vi "Compact.vi"(1 "bytestream":refnum<class "Bytestream.lvclass">) -> (0 "bytestream out":refnum<class "Bytestream.lvclass">)   [LabVIEW 2020, in "NI_Bytestream.lvlib" / "Bytestream.lvclass"]
uses:
  <vilib>/Array/Bytestream/Bytestream.lvclass
  <vilib>/Array/Bytestream/Bytestream.lvclass/Bytestream.ctl
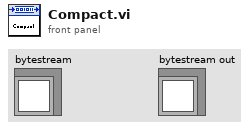
[diagram p1: front panel]
types:
  T1 = typedef "NI_Bytestream.lvlib/Bytestream.lvclass/Datum.ctl" = cluster{"array":u8[], "index":i32}
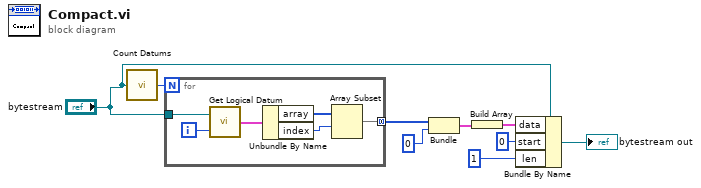
[diagram p0: block diagram]
diagram:
  n1 = call <vilib>:"Count Datums.vi"("bytestream"="bytestream") -> ("datums"=w6:i32)
  n2 = for {
    N: w6 -> [_]
    tunnel: "bytestream" -> [w15]
    tunnel: [w10] -> w5 mode=concatenating
    i -> [w14]
    n3 = call <vilib>:"Get Logical Datum.vi"("index"=w14, "bytestream"=w15) -> ("datum"=w13:T1)
    n4 = Unbundle By Name(w13) -> ("array"=w12:u8[], "index"=w11:i32)
    n5 = Array Subset(array=w12, index=w11) -> (w10:u8[])  [unwired: 1 in]
  }
  n6 = Bundle(w5, 0) -> (w8:cluster{u8[], i32})  [unwired: 1 in]
  n7 = Build Array(w8) -> (w4:cluster{u8[], i32}[])
  n8 = Bundle By Name(cluster="bytestream", "data"=w4, "start"=0, "len"=1) -> (→"bytestream out":refnum<class "Bytestream.lvclass">)
